vi "Enable Low Charge Injection Mode.vi"(8 "error in (no error)":errorcluster, 10 "Enable Low Charge Injection Mode (F: Disable)":bool, 11 "VISA resource name":refnum<visa-resource-name>) -> (0 "error out":errorcluster, 3 "VISA resource name out":refnum<visa-resource-name>)   [LabVIEW 2021, in "Keithley 2182.lvlib"]
doc: "Enables or Disables instrument's Low Charge Injection Mode (pumpout current).\n\nIf you must use Channel 2 for measurements below 1V and the impedance between Channel 2 LO and Channel 1 LO is >100 uOhms, you can enable the Low Charge Injection Mode to reduce the pumpout current. However, this mode increases measurement noise by up to 8 times."
uses:
  <instrlib>/Keithley 2182/Keithley 2182.lvlib
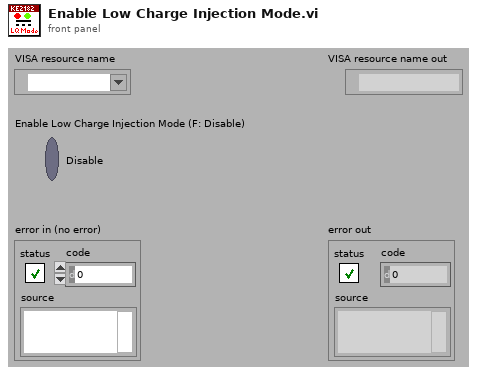
[diagram p1: front panel]
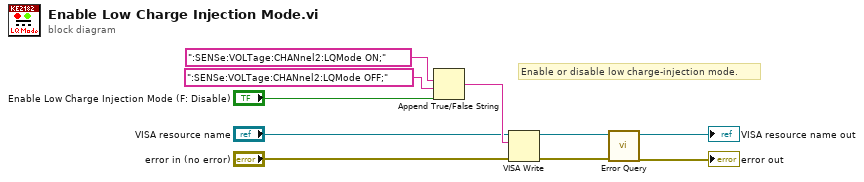
[diagram p0: block diagram]
diagram:
  # "Enable or disable low charge-injection mode."
  n1 = Append True/False String(1:"Enable Low Charge Injection Mode (F: Disable)", 2:":SENSe:VOLTage:CHANnel2:LQMode OFF;", 3:":SENSe:VOLTage:CHANnel2:LQMode ON;") -> (0:w7:string)  [unwired: 1 in]
  n2 = VISA Write(VISA resource name="VISA resource name", write buffer=w7, error in (no error)="error in (no error)") -> (VISA resource name out=w4:refnum<visa-resource-name>, error out=w3:errorcluster)  [unwired: 1 out]
  n3 = call <instrlib>:"Error Query.vi"("error in (no error)"=w3, "VISA resource name"=w4) -> ("error out"=→"error out":errorcluster, "VISA resource name out"=→"VISA resource name out":refnum<visa-resource-name>)  [unwired: 6 in, 2 out]
